vi "Pololu.Deg to us and Pololu Value Converter.vi"(7 "us to Units Mult":dbl=4.0, 9 "Set Pos (Deg)":dbl(slide) max=270.0 scale=0.0..270.0 scale format="%.1f", 11 "Range Info":T1={"Min us"=500.0, "Max us"=2500.0, "Min deg"=0.0, "Max deg"=270.0, "LStopDeg"=0.0, "UStopDeg"=270.0}) -> (1 "Cmd units":u16, 3 "Cmd us":dbl format="%.1f")   [LabVIEW 2018]
uses:
  Pololu.Device Range Config.ctl
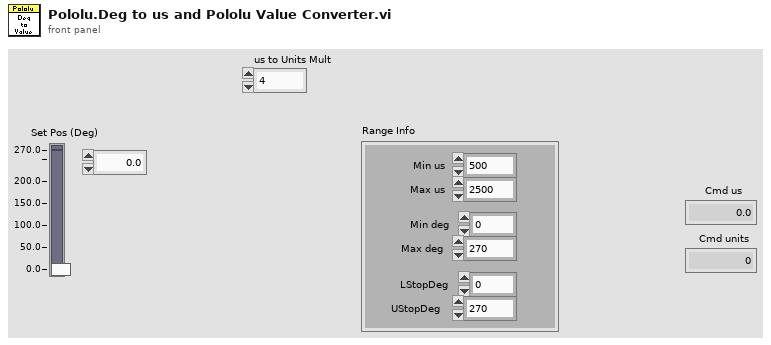
[diagram p1: front panel]
types:
  T1 = typedef "Pololu.Device Range Config.ctl" = cluster{"Min us":dbl, "Max us":dbl, "Min deg":dbl, "Max deg":dbl, "LStopDeg":dbl, "UStopDeg":dbl}
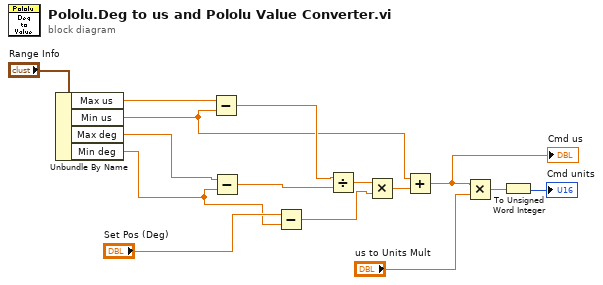
[diagram p0: block diagram]
diagram:
  n1 = Unbundle By Name("Range Info") -> ("Max us"=w3:dbl, "Min us"=w2:dbl, "Max deg"=w5:dbl, "Min deg"=w4:dbl)
  n2 = Subtract(x=w3, y=w2) -> (x-y=w13:dbl)
  n3 = Subtract(x=w5, y=w4) -> (x-y=w12:dbl)
  n4 = Subtract(x="Set Pos (Deg)", y=w4) -> (x-y=w10:dbl)
  n5 = Divide(x=w13, y=w12) -> (x/y=w11:dbl)
  n6 = Multiply(x=w11, y=w10) -> (x*y=w9:dbl)
  n7 = Add(x=w2, y=w9) -> (x+y=w8:dbl)
  "Cmd us" <- w8
  n8 = Multiply(x=w8, y="us to Units Mult") -> (x*y=w7:dbl)
  n9 = To Unsigned Word Integer(number=w7) -> (unsigned 16bit integer=→"Cmd units":u16)
